vi "convertCurrentUnitsToEncoderUnits.vi"(8 "error in (no error)":errorcluster, 10 "Value In Current Units":dbl, 11 "Axis in":refnum<class "Axis.lvclass">) -> (0 "error out":errorcluster, 2 "Value In Encoder Units":i32, 3 "Axis out":refnum<class "Axis.lvclass">)   [LabVIEW 2019, in "Axis.lvclass"]
uses:
  Axis.lvclass
  Axis.lvclass/Axis.ctl
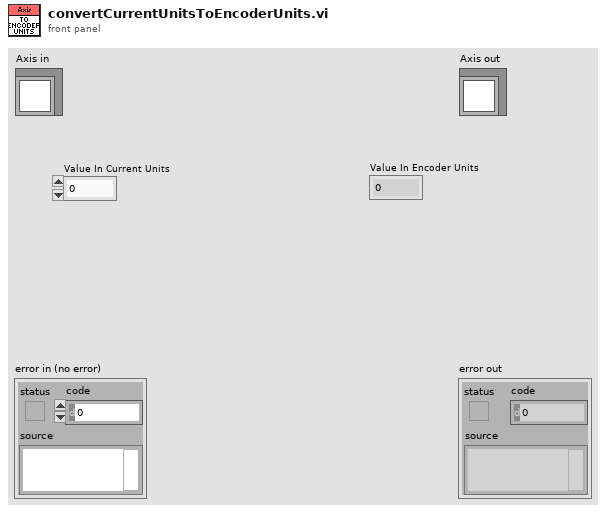
[diagram p1: front panel]
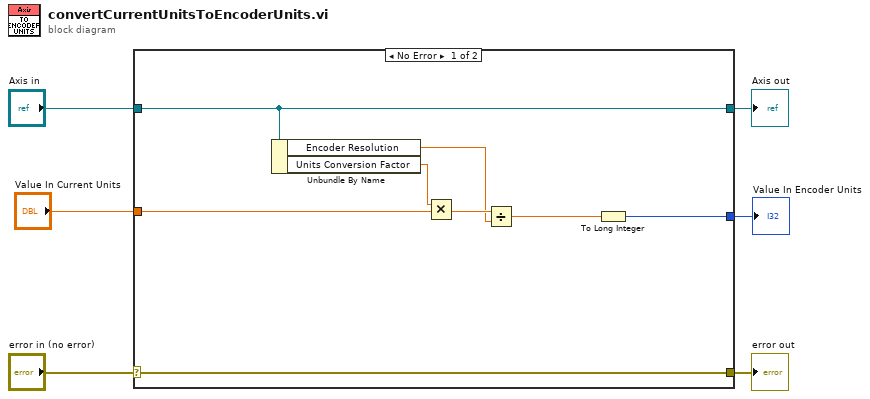
[diagram p0: block diagram]
diagram:
  n1 = case shown="No Error" "error in (no error)" {
    selector: "error in (no error)" -> [w14 w16]
    tunnel: [w14 w16] -> w5
    tunnel: [w10 w15] -> w3
    tunnel: "Axis in" -> [w10 w15]
    tunnel: [w7 _] -> w2
    tunnel: "Value In Current Units" -> [w8 _]
    frame No Error {
      n2 = Unbundle By Name(w10) -> ("Encoder Resolution"=w11:dbl, "Units Conversion Factor"=w13:dbl)
      n3 = Multiply(x=w13, y=w8) -> (x*y=w12:dbl)
      n4 = Divide(x=w12, y=w11) -> (x/y=w9:dbl)
      n5 = To Long Integer(number=w9) -> (32bit integer=w7:i32)
    }
    frame Error {
    }
  }
  "error out" <- w5
  "Axis out" <- w3
  "Value In Encoder Units" <- w2
